vi "API BARQUIT.vi"   [LabVIEW 2011, in "API READBC.lvlib"]
uses:
  API READBC.lvlib
  BarCodeAPI.dll
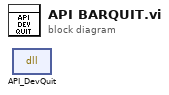
[diagram p0: block diagram]
diagram:
  n1 = dll-call lib="PTH1oabs CUsers\nAdministratorDesktop可重构机电平台项目DemoLabView基础APIBarCodeAPI.dll" fn="API_DevQuit"() -> ()  [unwired: 4 in, 2 out]
